vi "MAG3110_Read.vi"(0 "VISA resource name":refnum<visa-resource-name>, 11 "error in (no error)":errorcluster) -> (4 "VISA resource name out":refnum<visa-resource-name>, 6 "X (uT)":dbl, 8 "Y (uT)":dbl, 10 "Z (uT)":dbl, 15 "error out":errorcluster)   [LabVIEW 2012]
panel:
  out "substring":string
  out "read buffer 2":string
  out "read buffer":string
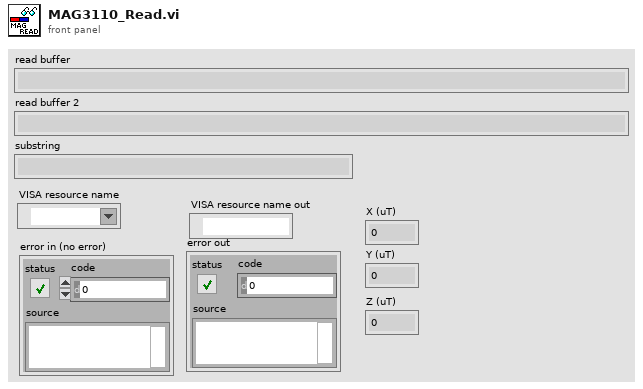
[diagram p1: front panel]
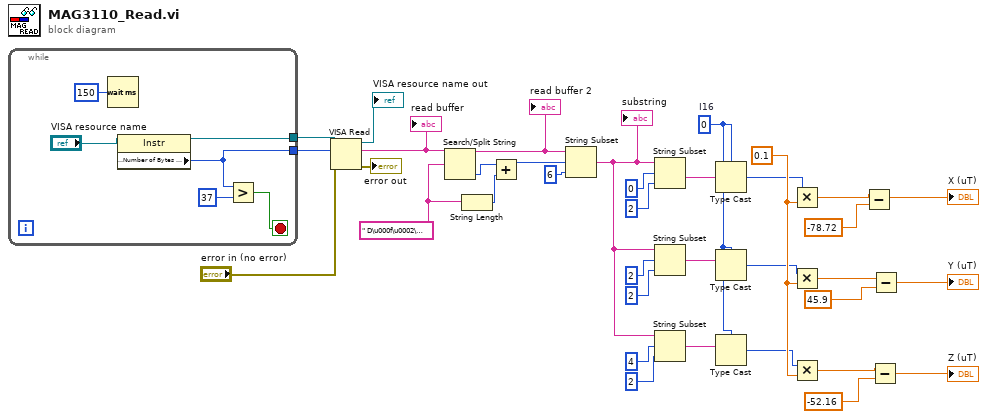
[diagram p0: block diagram]
diagram:
  w14 = i16 0  # I16
  w20 = 0.1
  w29 = " D\u000f\u0002\u0001" ("search string/char (-)")
  n1 = while {
    tunnel: [w39] -> w2
    tunnel: [w38] -> w1
    stop <- w37 stop-if-true
    n2 = Wait (ms)(milliseconds to wait=u32 150) -> ()  [unwired: 1 out]
    n3 = property class="Instr"(reference="VISA resource name") -> (reference out=w39:refnum<visa-resource-name>, "Serial Settings:Number of Bytes at Serial Port"=w38:u32)  [unwired: 1 in, 1 out]
    n4 = Greater?(x=w38, y=u32 37) -> (0:w37:bool)
  }
  n5 = VISA Read(VISA resource name=w2, byte count=w1, error in (no error)="error in (no error)") -> (VISA resource name out=→"VISA resource name out":refnum<visa-resource-name>, read buffer=w33:string, error out=→"error out":errorcluster)  [unwired: 1 out]
  "read buffer" <- w33
  "read buffer 2" <- w33
  n6 = Search/Split String(string=w33, search string/char (-)=w29) -> (offset of match=w32:i32)  [unwired: 1 in, 2 out]
  n7 = String Length(string=w29) -> (length=w30:i32)
  n8 = Add(x=w32, y=w30) -> (x+y=w31:i32)
  n9 = String Subset(string=w33, offset (0)=w31, length (rest)=6 ("length (rest)")) -> (substring=w21:string)
  "substring" <- w21
  n10 = String Subset(string=w21, offset (0)=0, length (rest)=2 ("length (rest)")) -> (substring=w19:string)
  n11 = String Subset(string=w21, offset (0)=2, length (rest)=2 ("length (rest)")) -> (substring=w16:string)
  n12 = String Subset(string=w21, offset (0)=4, length (rest)=2 ("length (rest)")) -> (substring=w15:string)
  n13 = Type Cast(type=w14, x=w19) -> (*(type *) &x=w17:i16)
  n14 = Type Cast(type=w14, x=w16) -> (*(type *) &x=w12:i16)
  n15 = Type Cast(type=w14, x=w15) -> (*(type *) &x=w13:i16)
  n16 = Multiply(x=w17, y=w20) -> (x*y=w10:dbl)
  n17 = Multiply(x=w12, y=w20) -> (x*y=w8:dbl)
  n18 = Multiply(x=w13, y=w20) -> (x*y=w5:dbl)
  n19 = Subtract(x=w10, y=-78.72) -> (x-y=→"X (uT)":dbl)
  n20 = Subtract(x=w5, y=-52.16) -> (x-y=→"Z (uT)":dbl)
  n21 = Subtract(x=w8, y=45.9) -> (x-y=→"Y (uT)":dbl)
